vi "GLBL -GPSLocation.vi"() -> ()   [LabVIEW 2019]
panel:
  out "EXIT-GPS":bool
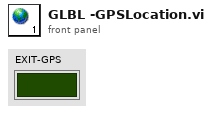
[diagram p1: front panel]
diagram:
